vi "PhidgetOpen.vi"(5 "IsHubPort":bool, 8 "error in":errorcluster, 9 "millis":i32=5000, 10 "Phidget ID":u64=18446744073709551615, 11 "Device Info":T1={"Serial Number"=-1, "Channel"=0, "Port"=0}) -> (0 "error out":errorcluster, 1 "Attached?":bool, 2 "Serial Number Return":i32, 3 "Device Out":u64)   [LabVIEW 2012, in "Phidget Common.lvlib"]
doc: "${Open:Header}"
uses:
  <instrlib>/Phidgets/Phidget Common/Phidget Common.lvlib
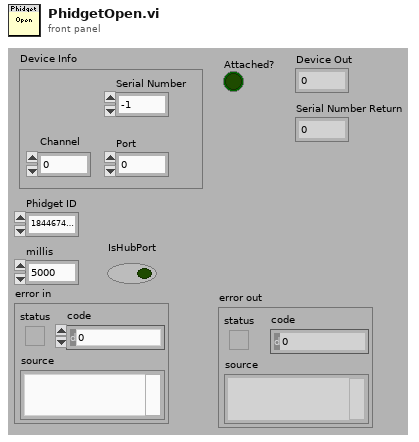
[diagram p1: front panel]
types:
  T1 = cluster{"Serial Number":i32, "Channel":i32, "Port":i32}
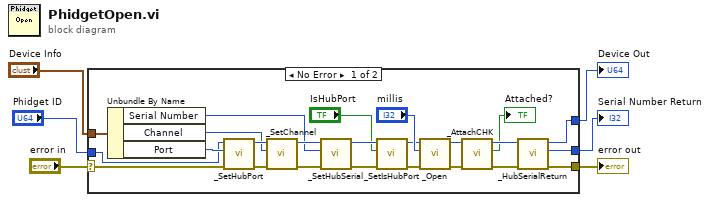
[diagram p0: block diagram]
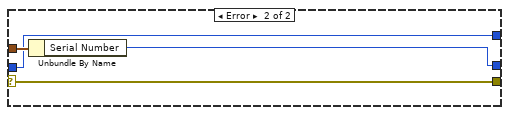
[diagram p2: hidden frame]
diagram:
  n1 = case shown="No Error" "error in" {
    selector: "error in" -> [w19 w34]
    tunnel: [w29 w34] -> w5
    tunnel: "Device Info" -> [w15 w32]
    tunnel: [w14 w31] -> w3
    tunnel: [w13 w33] -> w2
    tunnel: "Phidget ID" -> [w12 w31]
    frame No Error {
      n2 = Unbundle By Name(w15) -> ("Serial Number"=w18:i32, "Channel"=w17:i32, "Port"=w16:i32)
      n3 = call <instrlib>:"_SetHubPort.vi"("error in"=w19, "HubPort"=w16, "Device In"=w12) -> ("error out"=w22:errorcluster, "Device Out"=w23:u64)  [unwired: 7 in]
      n4 = call <instrlib>:"_SetChannel.vi"("error in"=w22, "Channel"=w17, "Device In"=w23) -> ("error out"=w20:errorcluster, "Device Out"=w21:u64)  [unwired: 7 in]
      n5 = call <instrlib>:"_SetHubSerial.vi"("error in"=w20, "HubSerial"=w18, "Device In"=w21) -> ("error out"=w11:errorcluster, "Device Out"=w10:u64)  [unwired: 7 in]
      n6 = call <instrlib>:"_SetIsHubPort.vi"("error in"=w11, "IsHubPort"="IsHubPort", "Device In"=w10) -> ("error out"=w8:errorcluster, "Device Out"=w9:u64)  [unwired: 7 in]
      n7 = call <instrlib>:"_Open.vi"("error in"=w8, "Timeout (mSec)"="millis", "Device In"=w9) -> ("error out"=w24:errorcluster, "Device Out"=w25:u64)  [unwired: 7 in]
      n8 = call <instrlib>:"_AttachCHK.vi"("error in"=w24, "Device In"=w25) -> ("error out"=w30:errorcluster, "Attached?"=→"Attached?":bool, "Device Out"=w28:u64)  [unwired: 7 in]
      n9 = call <instrlib>:"_HubSerialReturn.vi"("error in"=w30, "Device In"=w28) -> ("error out"=w29:errorcluster, "Serial Number Return"=w13:i32, "Device Out"=w14:u64)  [unwired: 7 in]
    }
    frame Error {
      n10 = Unbundle By Name(w32) -> ("Serial Number"=w33:i32)
    }
  }
  "error out" <- w5
  "Device Out" <- w3
  "Serial Number Return" <- w2
